vi "mxwScript_API_XMLWireToNodeByName.vi"(8 "error in (no error)":errorcluster, 10 "terminalName":string, 11 "nodeLabel":string) -> (0 "error out":errorcluster, 3 "encoded connector name":string)   [LabVIEW 2020]
doc: "Create encoded control name for connecting to a terminal on a generic node instead of to a control terminal. Terminal is specified by name. If multiple terminals with the same name exist, the first one is used.\n\nThis encoding works for both connected to and connected from terminals."
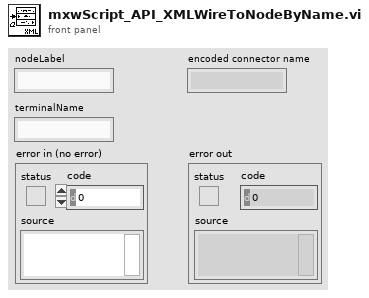
[diagram p1: front panel]
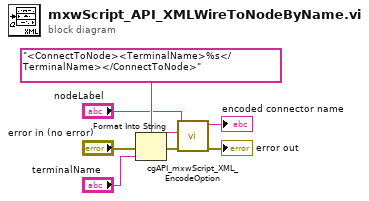
[diagram p0: block diagram]
diagram:
  n1 = Format Into String(format string="<ConnectToNode><TerminalName>%s</TerminalName></ConnectToNode>" ("control name"), error in="error in (no error)", "terminalName") -> (resulting string=w4:string, error out=w6:errorcluster)  [unwired: 1 in]
  n2 = call "cgAPI_mxwScript_XML_EncodeOption.vi"("error in (no error)"=w6, "otherXML"=w4, "normalTextString"="nodeLabel") -> ("error out"=→"error out":errorcluster, "encodedString"=→"encoded connector name":string)  [unwired: 7 out]
